vi "IoT VIs.vi"() -> ()   [LabVIEW 2019]
uses:
  <vilib>/httpClient/LabVIEWHTTPClient.lvlib
  <vilib>/httpClient/POSTBuffer.vi
  <vilib>/httpClient/PUTBuffer.vi
  EN1Course-master/_Subs/ThingWorx/_TW_Subs/Thingworx_Write_Bool.vi
  EN1Course-master/_Subs/SystemLink/SL_Subs/SystemLink_Write_Boolean.vi
  EN1Course-master/_Subs/OpenDiagram/Open_XControl.xctl
panel:
  in  "OpenDiag":refnum<vi>(xcontrol)
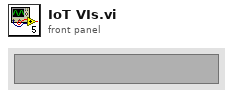
[diagram p1: front panel]
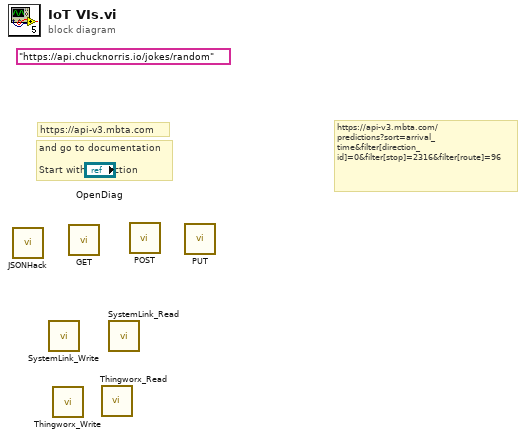
[diagram p0: block diagram]
diagram:
  (unwired) "https://api.chucknorris.io/jokes/random"
  # "https://api-v3.mbta.com/predictions?sort=arrival_time&filter[direction_id]=0&filter[stop]=2316&filter[route]=96"
  # "and go to documentation\n\nStart with prediction"
  # "https://api-v3.mbta.com"
  n1 = call "JSONHack.vi"() -> ()  [unwired: 8 in, 4 out]
  n2 = call-poly "SystemLink_Write.vi"() -> ()  [unwired: 12 in]
  n3 = call-poly "Thingworx_Write.vi"() -> ()  [unwired: 12 in]
  n4 = call <vilib>:"GET.vi"() -> ()  [unwired: 12 in, 4 out]
  n5 = call "Thingworx_Read.vi"() -> ()  [unwired: 10 in, 2 out]
  n6 = call "SystemLink_Read.vi"() -> ()  [unwired: 9 in, 3 out]
  n7 = call-poly <vilib>:"POST.vi"() -> ()  [unwired: 12 in, 4 out]
  n8 = call-poly <vilib>:"PUT.vi"() -> ()  [unwired: 12 in, 4 out]
